vi "movestage.vi"   [LabVIEW 2015]
uses:
  <vilib>/Instr/_visa.llb/VISA Configure Serial Port (Instr).vi
types:
  T1 = cluster{"upleft":bool, "up":bool, "upright":bool, "right":bool, "downright":bool, "down":bool, "downleft":bool, "left":bool, "Bigsmall":bool, "E_stage":errorcluster}
  T2 = cluster{"StageS":i32, "StageL":i32, "currmeas data dir":path, "image OD":u16, "contour OD":u16, "point OD":u16, "AOlines":tag[], "AIlines":tag[], "CI lines":tag[], "DO lines":tag[], "AO names":string[], "CI names":string[], "AI names":string[], "DO names":string[], "CIextensions":string[], "AIextensions":string[], "Voltage to Ygalvo":i32, "Voltage to Xgalvo":i32, "Voltage to patch":i32, "640 shutter":i32, "2P shutter":i32, "LT timestamp":u32, "Vp":i32, "Ip":i32, "camera trigger":i32, "master data dir":path, "voltage to Zpos":i32, "Vto2P":i32, "640 AO":i32, "488 AO":i32, "532 AO":i32, "640TTL":u32, "488TTL":u32, "532TTL":u32, "Device 1 sampleclock out":tag, "Device 1 Starttrigger out":tag, "Device 2 sampleclock in":tag, "Device 2 StartTrigger in ":tag, "2PODTTL":u32, "488 shutter":u32, "LCVR red":u32, "LCVR blue":u32}
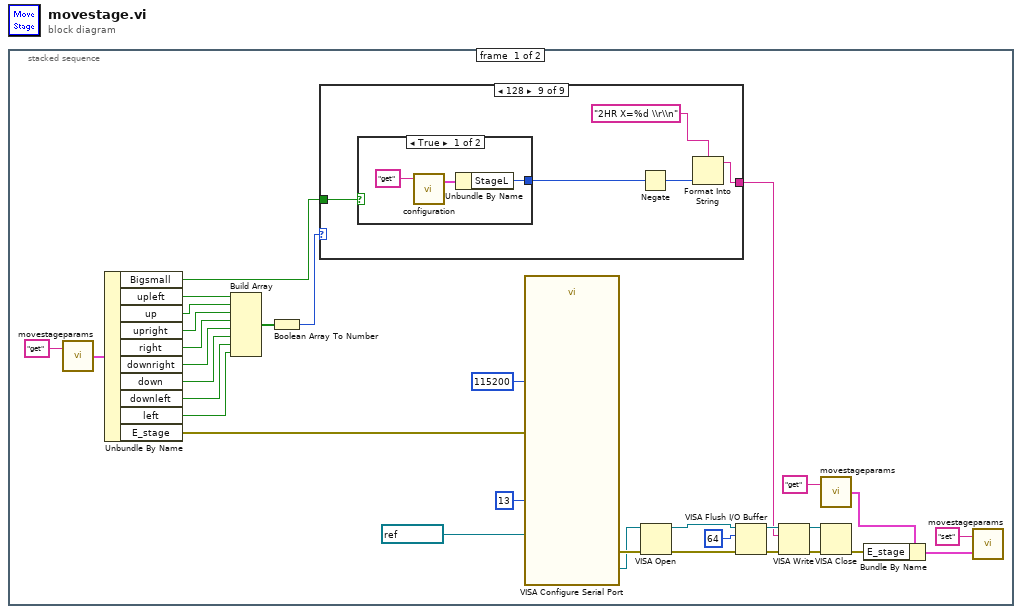
[diagram p0: block diagram]
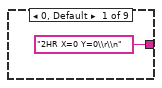
[diagram p2: hidden frame]
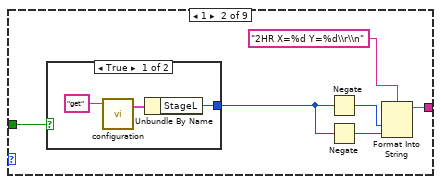
[diagram p3: hidden frame]
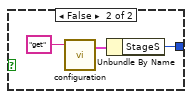
[diagram p4: hidden frame]
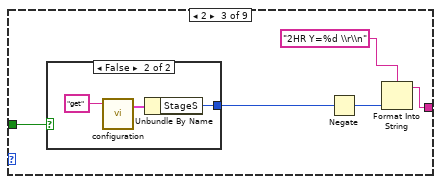
[diagram p5: hidden frame]
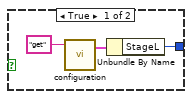
[diagram p6: hidden frame]
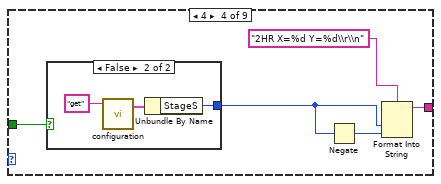
[diagram p7: hidden frame]
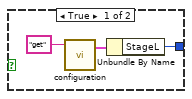
[diagram p8: hidden frame]
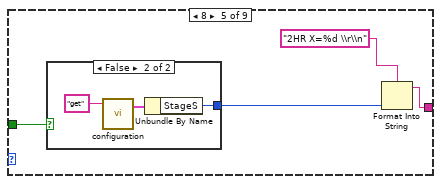
[diagram p9: hidden frame]
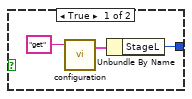
[diagram p10: hidden frame]
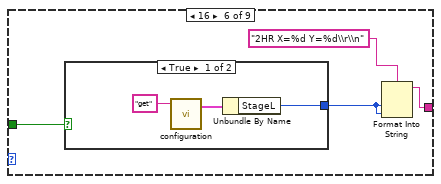
[diagram p11: hidden frame]
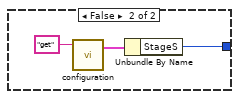
[diagram p12: hidden frame]
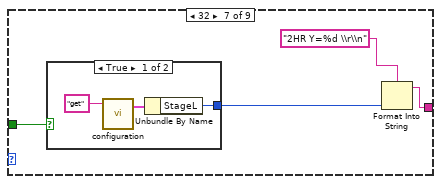
[diagram p13: hidden frame]
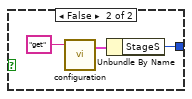
[diagram p14: hidden frame]
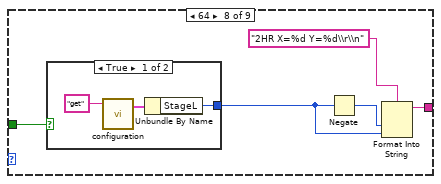
[diagram p15: hidden frame]
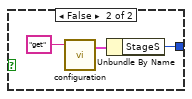
[diagram p16: hidden frame]
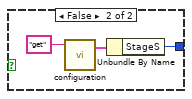
[diagram p17: hidden frame]
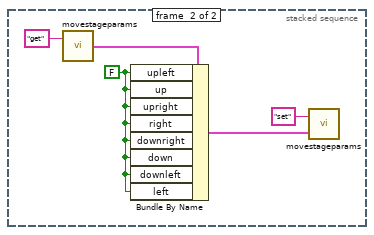
[diagram p18: hidden frame]
diagram:
  n1 = stacked-sequence {
    frame #0 {
      n2 = call "movestageparams.vi"("command"="get") -> ("Params out"=w17:T1)  [unwired: 1 in]
      n3 = Unbundle By Name(w17) -> ("Bigsmall"=w26:bool, "upleft"=w18:bool, "up"=w19:bool, "upright"=w20:bool, "right"=w21:bool, "downright"=w22:bool, "down"=w23:bool, "downleft"=w24:bool, "left"=w25:bool, "E_stage"=w27:errorcluster)
      n4 = Build Array(w18, w19, w20, w21, w22, w23, w24, w25) -> (w14:bool[])
      n5 = Boolean Array To Number(Boolean array=w14) -> (number=w15:u32)
      n6 = case shown="128" w15 {
        tunnel: ["2HR X=0 Y=0\\r\\n" w35 w49 w58 w69 w79 w89 w99 w110] -> w3
        tunnel: w26 -> [_ w34 w46 w57 w68 w78 w88 w98 w109]
        frame 0, Default {
        }
        frame 1 {
          n7 = case shown="True" w34 {
            tunnel: [w40 w43] -> w37
            frame True {
              n8 = call "configuration.vi"("command"="get") -> ("config out"=w41:T2)  [unwired: 2 in, 1 out]
              n9 = Unbundle By Name(w41) -> ("StageL"=w40:i32)
            }
            frame False {
              n10 = call "configuration.vi"("command"="get") -> ("config out"=w44:T2)  [unwired: 2 in, 1 out]
              n11 = Unbundle By Name(w44) -> ("StageS"=w43:i32)
            }
          }
          n12 = Negate(x=w37) -> (-x=w38:i32)
          n13 = Negate(x=w37) -> (-x=w39:i32)
          n14 = Format Into String(format string="2HR X=%d Y=%d\\r\\n", w38, w39) -> (resulting string=w35:string)  [unwired: 2 in, 1 out]
        }
        frame 2 {
          n15 = case shown="False" w46 {
            tunnel: [w51 w54] -> w48
            frame True {
              n16 = call "configuration.vi"("command"="get") -> ("config out"=w52:T2)  [unwired: 2 in, 1 out]
              n17 = Unbundle By Name(w52) -> ("StageL"=w51:i32)
            }
            frame False {
              n18 = call "configuration.vi"("command"="get") -> ("config out"=w55:T2)  [unwired: 2 in, 1 out]
              n19 = Unbundle By Name(w55) -> ("StageS"=w54:i32)
            }
          }
          n20 = Negate(x=w48) -> (-x=w47:i32)
          n21 = Format Into String(format string="2HR Y=%d \\r\\n", w47) -> (resulting string=w49:string)  [unwired: 2 in, 1 out]
        }
        frame 4 {
          n22 = case shown="False" w57 {
            tunnel: [w62 w65] -> w60
            frame True {
              n23 = call "configuration.vi"("command"="get") -> ("config out"=w63:T2)  [unwired: 2 in, 1 out]
              n24 = Unbundle By Name(w63) -> ("StageL"=w62:i32)
            }
            frame False {
              n25 = call "configuration.vi"("command"="get") -> ("config out"=w66:T2)  [unwired: 2 in, 1 out]
              n26 = Unbundle By Name(w66) -> ("StageS"=w65:i32)
            }
          }
          n27 = Negate(x=w60) -> (-x=w61:i32)
          n28 = Format Into String(format string="2HR X=%d Y=%d\\r\\n", w60, w61) -> (resulting string=w58:string)  [unwired: 2 in, 1 out]
        }
        frame 8 {
          n29 = case shown="False" w68 {
            tunnel: [w72 w75] -> w71
            frame True {
              n30 = call "configuration.vi"("command"="get") -> ("config out"=w73:T2)  [unwired: 2 in, 1 out]
              n31 = Unbundle By Name(w73) -> ("StageL"=w72:i32)
            }
            frame False {
              n32 = call "configuration.vi"("command"="get") -> ("config out"=w76:T2)  [unwired: 2 in, 1 out]
              n33 = Unbundle By Name(w76) -> ("StageS"=w75:i32)
            }
          }
          n34 = Format Into String(format string="2HR X=%d \\r\\n", w71) -> (resulting string=w69:string)  [unwired: 2 in, 1 out]
        }
        frame 16 {
          n35 = case shown="True" w78 {
            tunnel: [w82 w85] -> w81
            frame True {
              n36 = call "configuration.vi"("command"="get") -> ("config out"=w83:T2)  [unwired: 2 in, 1 out]
              n37 = Unbundle By Name(w83) -> ("StageL"=w82:i32)
            }
            frame False {
              n38 = call "configuration.vi"("command"="get") -> ("config out"=w86:T2)  [unwired: 2 in, 1 out]
              n39 = Unbundle By Name(w86) -> ("StageS"=w85:i32)
            }
          }
          n40 = Format Into String(format string="2HR X=%d Y=%d\\r\\n", w81, w81) -> (resulting string=w79:string)  [unwired: 2 in, 1 out]
        }
        frame 32 {
          n41 = case shown="True" w88 {
            tunnel: [w92 w95] -> w90
            frame True {
              n42 = call "configuration.vi"("command"="get") -> ("config out"=w93:T2)  [unwired: 2 in, 1 out]
              n43 = Unbundle By Name(w93) -> ("StageL"=w92:i32)
            }
            frame False {
              n44 = call "configuration.vi"("command"="get") -> ("config out"=w96:T2)  [unwired: 2 in, 1 out]
              n45 = Unbundle By Name(w96) -> ("StageS"=w95:i32)
            }
          }
          n46 = Format Into String(format string="2HR Y=%d \\r\\n", w90) -> (resulting string=w89:string)  [unwired: 2 in, 1 out]
        }
        frame 64 {
          n47 = case shown="True" w98 {
            tunnel: [w103 w106] -> w101
            frame True {
              n48 = call "configuration.vi"("command"="get") -> ("config out"=w104:T2)  [unwired: 2 in, 1 out]
              n49 = Unbundle By Name(w104) -> ("StageL"=w103:i32)
            }
            frame False {
              n50 = call "configuration.vi"("command"="get") -> ("config out"=w107:T2)  [unwired: 2 in, 1 out]
              n51 = Unbundle By Name(w107) -> ("StageS"=w106:i32)
            }
          }
          n52 = Negate(x=w101) -> (-x=w102:i32)
          n53 = Format Into String(format string="2HR X=%d Y=%d\\r\\n", w102, w101) -> (resulting string=w99:string)  [unwired: 2 in, 1 out]
        }
        frame 128 {
          n54 = case shown="True" w109 {
            tunnel: [w114 w117] -> w112
            frame True {
              n55 = call "configuration.vi"("command"="get") -> ("config out"=w115:T2)  [unwired: 2 in, 1 out]
              n56 = Unbundle By Name(w115) -> ("StageL"=w114:i32)
            }
            frame False {
              n57 = call "configuration.vi"("command"="get") -> ("config out"=w118:T2)  [unwired: 2 in, 1 out]
              n58 = Unbundle By Name(w118) -> ("StageS"=w117:i32)
            }
          }
          n59 = Negate(x=w112) -> (-x=w111:i32)
          n60 = Format Into String(format string="2HR X=%d \\r\\n", w111) -> (resulting string=w110:string)  [unwired: 2 in, 1 out]
        }
      }
      n61 = call-poly "VISA Configure Serial Port"("VISA resource name"=refnum<visa-resource-name> "COM1", "termination char\n(0xA = '\\n' = LF)"=u8 13 ("termination char\n(0xA = '\\n' = LF)"), "baud rate (9600)"=u32 115200 ("baud rate (9600) 2"), "error in (no error)"=w27) -> ("VISA resource name out"=w8:refnum<visa-resource-name>, "error out"=w12:errorcluster)  [unwired: 3 in, 7 out]
      n62 = VISA Open(error in (no error)=w12, VISA resource name=w8) -> (VISA resource name=w9:refnum<visa-resource-name>, error out=w13:errorcluster)  [unwired: 3 in]
      n63 = VISA Flush I/O Buffer(VISA resource name=w9, mask (16)=u16 64, error in (no error)=w13) -> (VISA resource name out=w4:refnum<visa-resource-name>, error out=w5:errorcluster)
      n64 = VISA Write(VISA resource name=w4, write buffer=w3, error in (no error)=w5) -> (VISA resource name out=w10:refnum<visa-resource-name>, error out=w11:errorcluster)  [unwired: 1 out]
      n65 = call "movestageparams.vi"("command"="get") -> ("Params out"=w30:T1)  [unwired: 1 in]
      n66 = VISA Close(VISA resource name=w10, error in (no error)=w11) -> (error out=w31:errorcluster)
      n67 = Bundle By Name(cluster=w30, "E_stage"=w31) -> (w32:T1)
      n68 = call "movestageparams.vi"("Params in"=w32, "command"="set") -> ()  [unwired: 1 out]
    }
    frame #1 {
      w121 = FALSE
      n69 = call "movestageparams.vi"("command"="get") -> ("Params out"=w122:T1)  [unwired: 1 in]
      n70 = Bundle By Name(cluster=w122, "upleft"=w121, "up"=w121, "upright"=w121, "right"=w121, "downright"=w121, "down"=w121, "downleft"=w121, "left"=w121) -> (w120:T1)
      n71 = call "movestageparams.vi"("Params in"=w120, "command"="set") -> ()  [unwired: 1 out]
    }
  }
